vi "FG GPS Data.vi"(1 "FG Action (Read)":T2, 2 "GPS Point in":T1) -> (0 "GPS Point out":T1)   [LabVIEW 2009]
uses:
  cRIO/Functional Global Variables/Actions for FG's.ctl
  Typedefs/EVS GPS Data.ctl
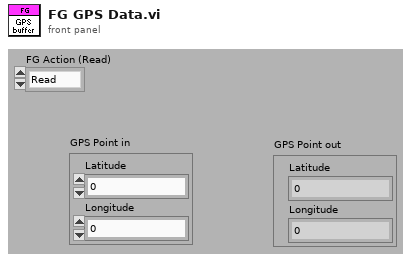
[diagram p1: front panel]
types:
  T1 = typedef "EVS GPS Data.ctl" = cluster{"Latitude":dbl, "Longitude":dbl}
  T2 = typedef "Actions for FG's.ctl" = enum16{"Read", "Write"}
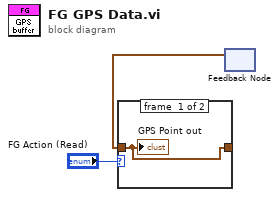
[diagram p0: block diagram]
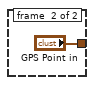
[diagram p2: hidden frame]
diagram:
  n1 = feedback #1() -> (w1:T1)  [unwired: 1 in]
  n2 = case shown="\"Read\", Default" "FG Action (Read)" {
    tunnel: [w4 "GPS Point in"] -> w2
    tunnel: w1 -> [w4 _]
    frame #0 {
      "GPS Point out" <- w4
    }
    frame #1 {
    }
  }
